vi "Optimizer-PB.vi"(10 "Optimize active channels":bool[](array[boolean])=[FALSE, FALSE, FALSE, TRUE], 11 "Optimize Parameters":T1={"Volt Step"={"X"=0.01, "Y"=0.01, "Z"=0.0}, "Num Iterations"=1, "Dwell Time (ms)"=100, "Volts Range"={"X"=0.1, "Y"=0.1, "Z"=0.0}, "Method"={"X"=enum."Max", "Y"=enum."Max", "Z"=enum."Max"}} {"Volts Range"."Z" min=0.0; "Volts Range"."Y" min=0.0; "Volts Range"."X" min=0.0; "Dwell Time (ms)" min=0; "Num Iterations" min=1 step=1; "Volt Step"."Z" min=1e-05; "Volt Step"."Y" min=1e-06; "Volt Step"."X" min=1e-06}) -> (2 "Final Counts/s":dbl, 3 "String":string)   [LabVIEW 2012]
uses:
  Strict Type Def - Optimize Parameters Cluster.ctl
  Channels.vi
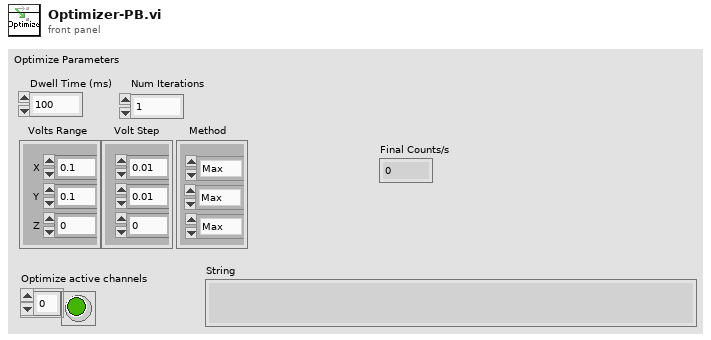
[diagram p1: front panel]
types:
  T1 = typedef "Strict Type Def - Optimize Parameters Cluster.ctl" = cluster{"Volt Step":cluster{"X":dbl, "Y":dbl, "Z":dbl}, "Num Iterations":i32, "Dwell Time (ms)":i32, "Volts Range":cluster{"X":dbl, "Y":dbl, "Z":dbl}, "Method":cluster{"X":enum16{"Max", "Gaussian"}, "Y":enum16{"Max", "Gaussian"}, "Z":enum16{"Max", "Gaussian"}}}
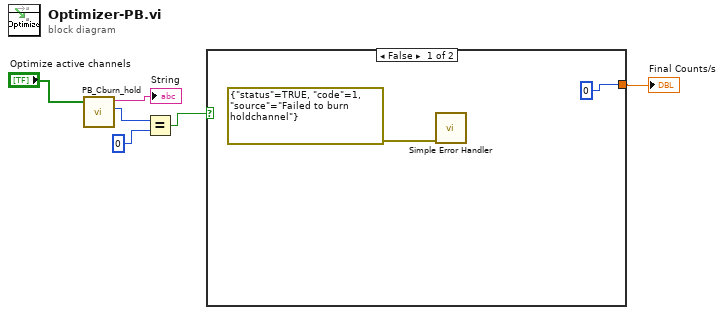
[diagram p0: block diagram]
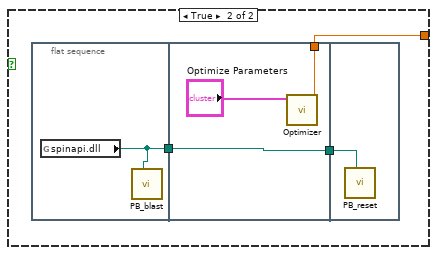
[diagram p2: hidden frame]
diagram:
  n1 = call "PB_Cburn_hold.vi"("Optimize active channels"="Optimize active channels") -> ("Return"=w4:i32, "String"=→"String":string)  [unwired: 9 in]
  n2 = Equal?(x=w4, y=0) -> (x = y?=w2:bool)
  n3 = case shown="False" w2 {
    tunnel: [0 w9] -> w1
    frame False {
      n4 = call <vilib>:"Simple Error Handler.vi"("error in (no error)"=errorcluster {"status"=TRUE, "code"=1, "source"="Failed to burn holdchannel"} ("error constant")) -> ()  [unwired: 4 in, 5 out]
    }
    frame True {
      n5 = flat-sequence {
        tunnel: [w12] -> w10
        tunnel: [w14] -> w11
        tunnel: w10 -> [w14]
        tunnel: [w13] -> w9
        tunnel: w11 -> [w16]
        frame #0 {
          n6 = global read "Channels.vi" "spinapi.dll"() -> (w12:path)
          n7 = call "PB_blast.vi"("Path to spinapi.dll"=w12) -> ()  [unwired: 7 in]
        }
        frame #1 {
          n8 = call "Optimizer.vi"("Optimize Parameters"="Optimize Parameters") -> ("Final Counts/s"=w13:dbl)  [unwired: 10 in]
        }
        frame #2 {
          n9 = call "PB_reset.vi"("Path to spinapi.dll"=w16) -> ()  [unwired: 7 in]
        }
      }
    }
  }
  "Final Counts/s" <- w1
